vi "Detecção de código.vi"() -> ()   [LabVIEW 2020]
panel:
  in  "Script Vision Assistant":enum16{"Teste 1", "Teste 2"}(ring)
  out "Frame Rate":dbl
  in  "Image Path":path=path "C:/gravação inusitta/Basler acA4024-29uc (23753420)_20210512_221707411_0001.tif"
  in  "Stop (F)":bool
  out "Image Out":T1(plugin-control)
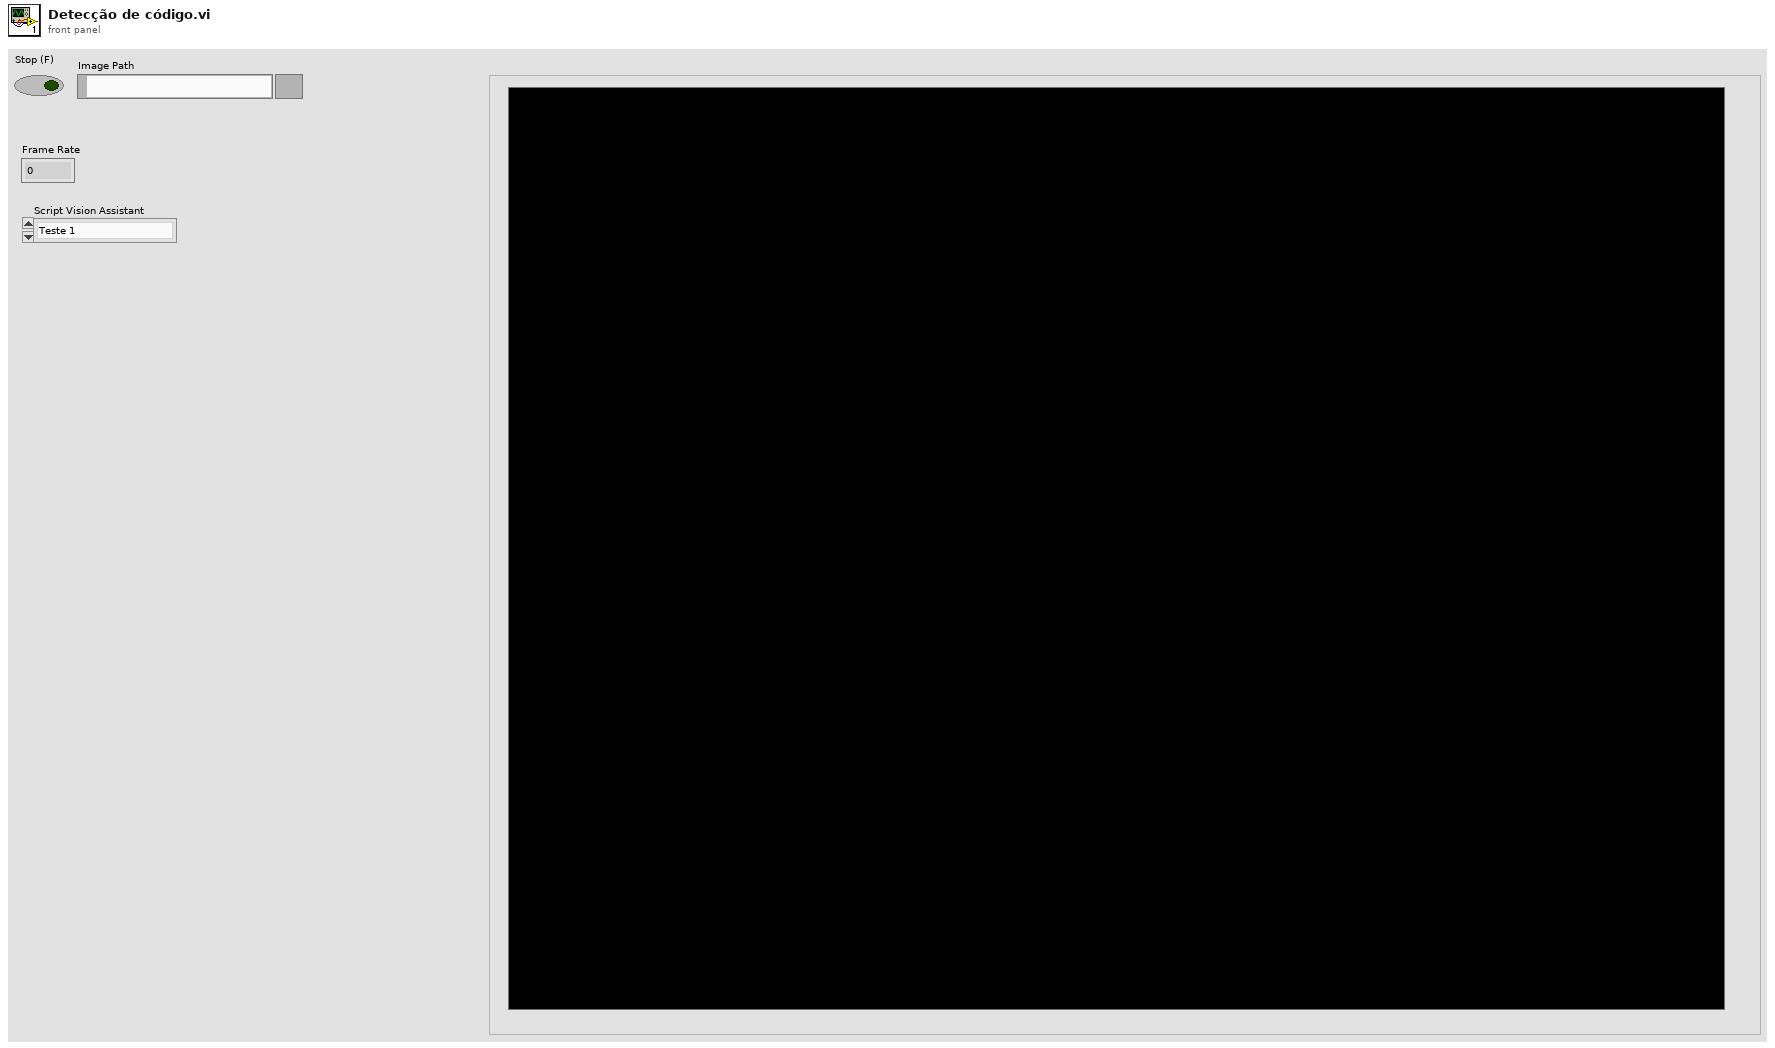
[diagram p1: front panel]
types:
  T1 = typedef "IMAQ Image.ctl" = refnum<image>
  T2 = cluster{"Desired Font (Application)":enum16{"User-specified Font", "Application Font", "System Font", "Dialog Font"}, "[User-specified Font]":cluster{"Font Name":string, "Size":i16, "Strikeout?":bool, "Italic?":bool, "Underline?":bool, "Outline?":bool, "Shadow?":bool, "Bold?":bool, "Rotation Angle":dbl}, "Horizontal Alignment":i16, "Vertical Alignment":i16}
  T3 = cluster{"Reference System":cluster{"Origin":cluster{"X":sgl, "Y":sgl}, "Angle (deg)":sgl, "Axis Reference":u32}, "Measurement System":cluster{"Origin":cluster{"X":sgl, "Y":sgl}, "Angle (deg)":sgl, "Axis Reference":u32}}
  T4 = typedef "QR Code Report.ctl" = cluster{"Found?":bool, "Data":string, "Bounding Box":cluster{"x":sgl, "y":sgl}[], "Errors Corrected":u32, "Dimensions (Rows/Cols)":u32, "Version":u32, "QR Model":T5, "Stream Mode":T6, "Barcode Polarity":T7, "Mirrored?":bool, "Append Stream Position":u32, "Size of Append Stream":u32, "First EAN-128 ID":i32, "First Alternate Language ID":i32, "Append Stream ID":u32, "Minimum Edge Strength":u32, "Demodulation Mode":T8, "Cell Sample Size":T9, "Cell Filter Mode":T10}
  T5 = typedef "QR Code Model Type.ctl" = i32
  T6 = typedef "QR Code Stream Mode Type.ctl" = i32
  T7 = typedef "Data Matrix Polarity.ctl" = i32
  T8 = typedef "Demodulation Mode.ctl" = i32
  T9 = typedef "Cell Sample Size.ctl" = i32
  T10 = typedef "Cell Filter Mode.ctl" = i32
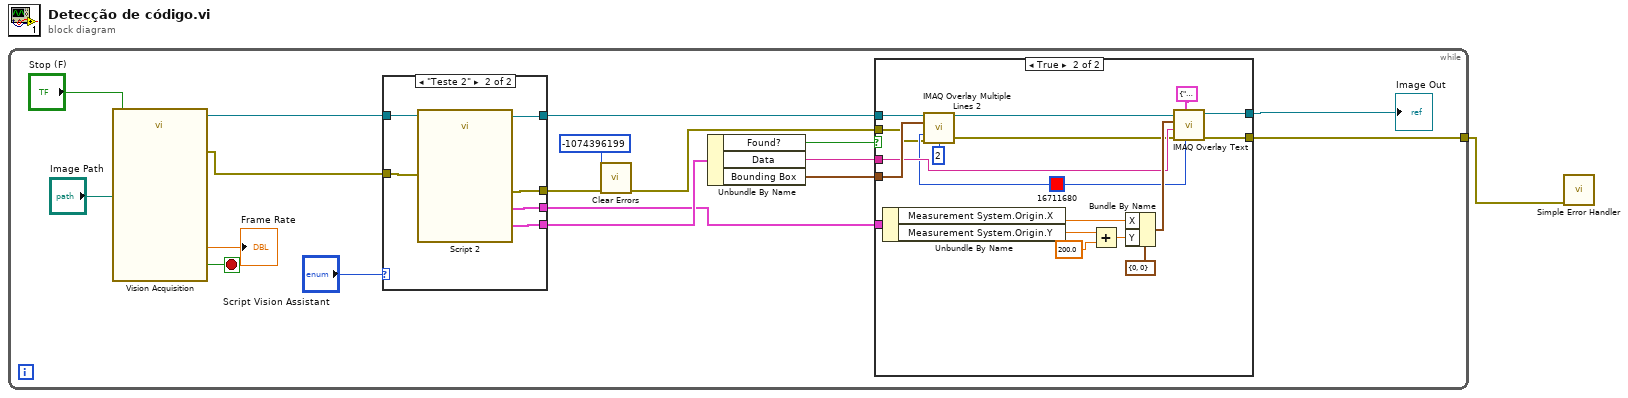
[diagram p0: block diagram]
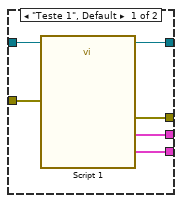
[diagram p2: hidden frame]
diagram:
  n1 = while {
    tunnel: [w6] -> w1
    stop <- w18 stop-if-true
    n2 = call "Vision Acquisition"("Image Path"="Image Path", "Stop (F)"="Stop (F)") -> ("Image Out"=w14:T1, "Frame Rate"=→"Frame Rate":dbl, "Stopped"=w18:bool, "error out"=w15:errorcluster)  [unwired: 21 in, 1 out]
    n3 = case shown="\"Teste 2\"" "Script Vision Assistant" {
      tunnel: w15 -> [w25 w29]
      tunnel: w14 -> [w24 w31]
      tunnel: [w23 w26] -> w13
      tunnel: [w22 w30] -> w10
      tunnel: [w21 w27] -> w8
      tunnel: [w20 w28] -> w5
      frame "Teste 1", Default {
        n4 = call "Script 1"("Image In"=w24, "error in"=w25) -> ("Image Out"=w22:T1, "Coordinate System Out (Coordenadas do provável QR Code)"=w21:T3, "QR Barcode Report (Leitura do código)"=w23:T4, "error out"=w20:errorcluster)  [unwired: 22 in]
      }
      frame "Teste 2" {
        n5 = call "Script 2"("Image In"=w31, "error in"=w29) -> ("Image Out"=w30:T1, "Coordinate System Out (Coordenadas do provável QR Code)"=w27:T3, "QR Barcode Report (Leitura do código)"=w26:T4, "error out"=w28:errorcluster)  [unwired: 22 in]
      }
    }
    n6 = call <vilib>:"Clear Errors.vi"("error in (no error)"=w5, "specific error code to clear (0: all)"=-1074396199) -> ("error out"=w4:errorcluster)  [unwired: 4 in, 1 out]
    n7 = Unbundle By Name(w13) -> ("Found?"=w12:bool, "Data"=w7:string, "Bounding Box"=w11:cluster{"x":sgl, "y":sgl}[])
    n8 = case shown="True" w12 {
      tunnel: w11 -> [_ w51]
      tunnel: w10 -> [w33 w50]
      tunnel: [w33 w47] -> w9
      tunnel: w8 -> [_ w46]
      tunnel: w7 -> [_ w39]
      tunnel: w4 -> [w32 w36]
      tunnel: [w32 w35] -> w6
      frame False {
      }
      frame True {
        w38 = u32 16711680 ("Color")
        n9 = Unbundle By Name(w46) -> ("Measurement System.Origin.X"=w44:sgl, "Measurement System.Origin.Y"=w42:sgl)
        n10 = call "IMAQ Overlay Multiple Lines 2"("Image"=w50, "Line End Points"=w51, "Color"=w38, "error in (no error)"=w36, "Width"=u32 2) -> ("Image Out"=w48:T1, "error out"=w37:errorcluster)  [unwired: 9 in]
        n11 = Add(x=w42, y=sgl 200.0) -> (x+y=w43:sgl)
        n12 = Bundle By Name(cluster=cluster{"X":i32, "Y":i32} {"X"=0, "Y"=0} ("Origin"), "X"=w44, "Y"=w43) -> (w40:cluster{"X":i32, "Y":i32})
        n13 = call "IMAQ Overlay Text"("Text Color (black)"=w38, "Font, Size & Style"=T2 {"Desired Font (Application)"=enum."User-specified Font", "[User-specified Font]"={"Font Name"="", "Size"=100, "Strikeout?"=FALSE, "Italic?"=FALSE, "Underline?"=FALSE, "Outline?"=FALSE, "Shadow?"=FALSE, "Bold?"=FALSE, "Rotation Angle"=0.0}, "Horizontal Alignment"=1, "Vertical Alignment"=0}, "error in (no error)"=w37, "String"=w39, "Origin"=w40, "Image"=w48) -> ("error out"=w35:errorcluster, "Image Out"=w47:T1)  [unwired: 4 in]
      }
    }
    "Image Out" <- w9
  }
  n14 = call <vilib>:"Simple Error Handler.vi"("error in (no error)"=w1) -> ()  [unwired: 4 in, 5 out]
